vi "show figure (SubVI).vi"(0 "y":bool, 1 "XYGraph引用句柄":refnum<vi>, 2 "文件名长度":i32, 3 "上次的数据列数":i32, 7 "新数据文件":path, 9 "Y输入":refnum<vi>, 12 "X输入":refnum<vi>, 14 "上一次的数据文件":path) -> (4 "figure2datafile输出":path, 6 "数值输出":i32)   [LabVIEW 2019, in "SubVI.lvlib"]
uses:
  SubVI.lvlib
  <vilib>/Utility/miscctls.llb/LVFormatAndPrecisionTypeDef.ctl
  <vilib>/Utility/file.llb/Read Delimited Spreadsheet (DBL).vi
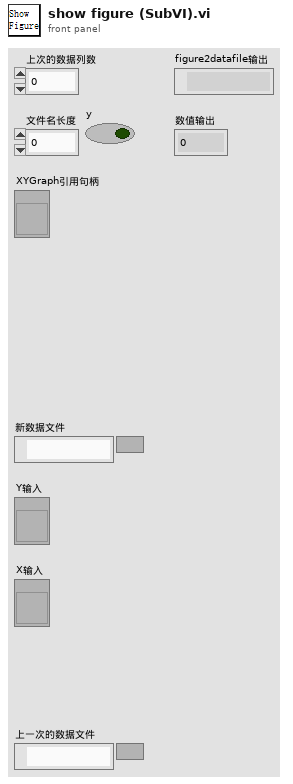
[diagram p1: front panel]
types:
  T1 = typedef "LVFormatAndPrecisionTypeDef.ctl" = cluster{"Format":u8, "Precision":u8}
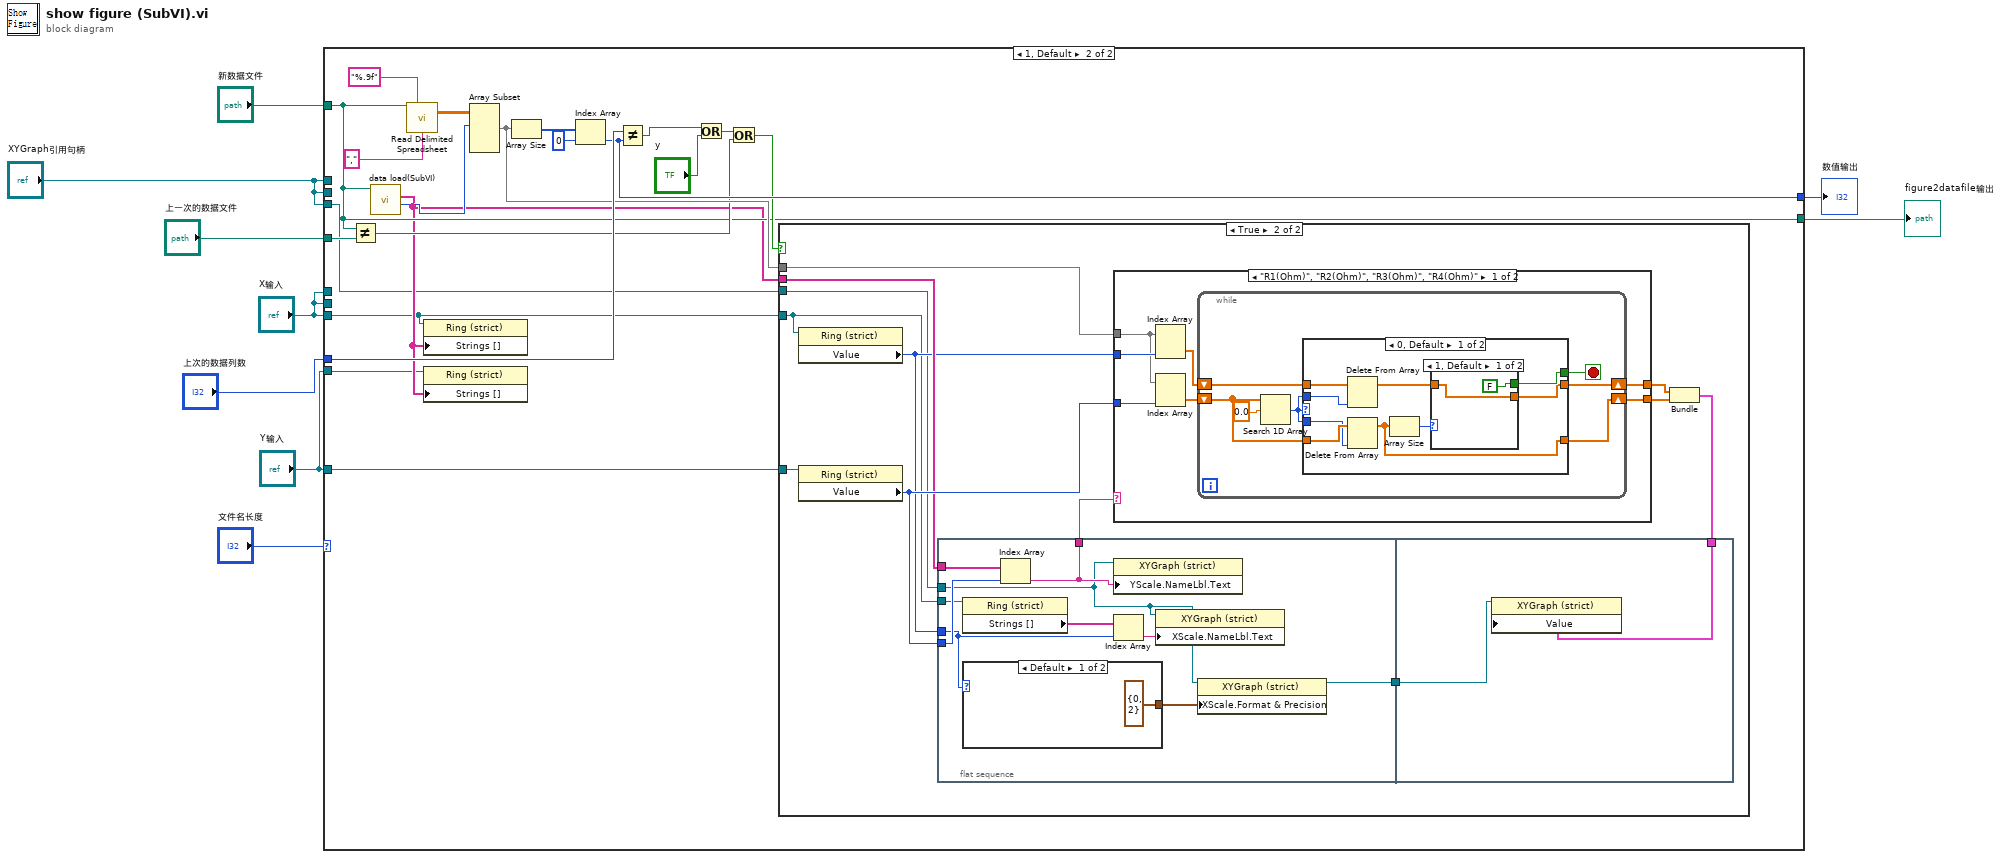
[diagram p0: block diagram]
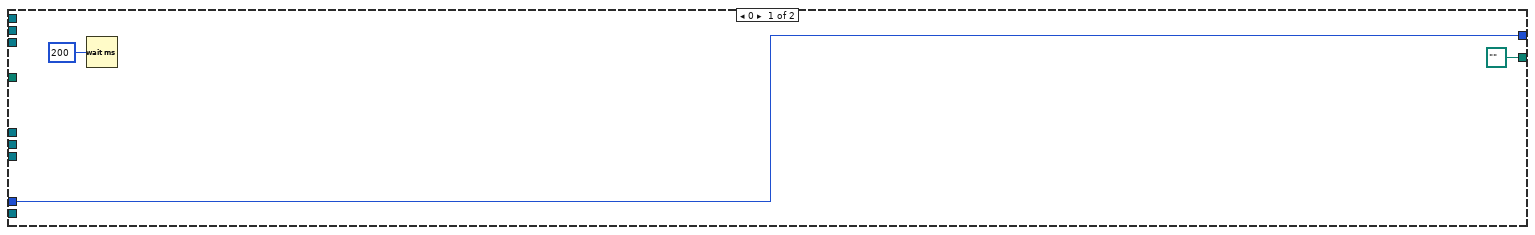
[diagram p2: hidden frame]
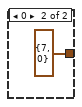
[diagram p4: hidden frame]
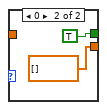
[diagram p5: hidden frame]
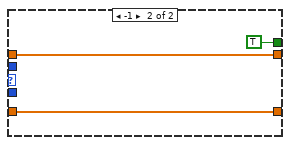
[diagram p6: hidden frame]
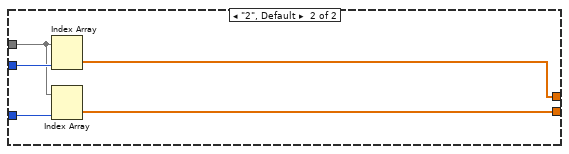
[diagram p7: hidden frame]
diagram:
  n1 = case shown="1, Default" "文件名长度" {
    tunnel: "新数据文件" -> [_ w21]
    tunnel: "上次的数据列数" -> [w12 w28]
    tunnel: [w12 w27] -> w7
    tunnel: "上一次的数据文件" -> [_ w25]
    tunnel: [path "" ("figure2datafile") w21] -> w9
    tunnel: "Y输入" -> [_ w18]
    tunnel: "X输入" -> [_ w14]
    tunnel: "X输入" -> [_ _]
    tunnel: "XYGraph引用句柄" -> [_ _]
    tunnel: "XYGraph引用句柄" -> [_ _]
    tunnel: "XYGraph引用句柄" -> [_ w16]
    tunnel: "X输入" -> [_ _]
    tunnel: "Y输入" -> [_ w15]
    frame 0 {
      n2 = Wait (ms)(milliseconds to wait=u32 200 ("等待时间（毫秒）")) -> ()  [unwired: 1 out]
    }
    frame 1, Default {
      n3 = Not Equal?(x=w21, y=w25) -> (x != y?=w23:bool)
      n4 = call "data load(SubVI).vi"("file path"=w21) -> ("数据起始行"=w20:i32, "项名"=w17:string[])  [unwired: 9 in]
      n5 = call-poly <vilib>:"Read Delimited Spreadsheet.vi"("file path (dialog if empty)"=w21, "format (%.3f)"="%.9f", "delimiter (\\t)"="," ("delimiter (\\t)")) -> ("all rows"=w33:dbl[][])  [unwired: 7 in, 5 out]
      n6 = property on="属性节点" class="Ring (strict)"(reference=w14, "Strings []"=w17) -> ()  [unwired: 1 in, 2 out]
      n7 = property on="属性节点" class="Ring (strict)"(reference=w15, "Strings []"=w17) -> ()  [unwired: 1 in, 2 out]
      n8 = Array Subset(array=w33, index (row)=w20) -> (w26:dbl[][])  [unwired: 3 in]
      n9 = Array Size(array=w26) -> (size(s)=w30:i32[])
      n10 = Index Array(array=w30, index=0 ("索引")) -> (element=w27:i32)
      n11 = Not Equal?(x=w28, y=w27) -> (x != y?=w31:bool)
      n12 = Or(x=w31, y="y") -> (x .or. y?=w24:bool)
      n13 = Or(x=w24, y=w23) -> (x .or. y?=w22:bool)
      n14 = case shown="True" w22 {
        tunnel: w26 -> [_ w42]
        tunnel: w18 -> [_ w40]
        tunnel: w17 -> [_ w38]
        tunnel: w14 -> [_ w35]
        tunnel: w16 -> [_ w36]
        frame False {
        }
        frame True {
          n15 = property class="Ring (strict)"(reference=w35) -> ("Value"=w37:u16)  [unwired: 1 in, 2 out]
          n16 = property class="Ring (strict)"(reference=w40) -> ("Value"=w39:u16)  [unwired: 1 in, 2 out]
          n17 = flat-sequence {
            tunnel: w37 -> [w51]
            tunnel: w39 -> [w52]
            tunnel: [w53] -> w41
            tunnel: w38 -> [w49]
            tunnel: w35 -> [w48]
            tunnel: w36 -> [w47]
            tunnel: [w46] -> w34
            tunnel: w44 -> [w58]
            tunnel: w34 -> [w59]
            frame #0 {
              n18 = property on="属性节点" class="Ring (strict)"(reference=w48) -> ("Strings []"=w55:string[])  [unwired: 1 in, 2 out]
              n19 = case shown="Default" w51 {
                tunnel: [T1 {"Format"=0, "Precision"=2} ("X标尺.显示格式") T1 {"Format"=7, "Precision"=0} ("X标尺.显示格式")] -> w50
                frame Default {
                }
                frame 0 {
                }
              }
              n20 = Index Array(array=w49, index=w52) -> (element=w53:string)
              n21 = property on="属性节点" class="XYGraph (strict)"(reference=w47, "YScale.NameLbl.Text"=w53) -> ()  [unwired: 1 in, 2 out]
              n22 = Index Array(array=w55, index=w51) -> (element=w54:string)
              n23 = property on="属性节点" class="XYGraph (strict)"(reference=w47, "XScale.NameLbl.Text"=w54) -> ()  [unwired: 1 in, 2 out]
              n24 = property on="属性节点" class="XYGraph (strict)"(reference=w47, "XScale.Format & Precision"=w50) -> (reference out=w46:refnum<vi>)  [unwired: 1 in, 1 out]
            }
            frame #1 {
              n25 = property on="属性节点" class="XYGraph (strict)"(reference=w59, "Value"=w58) -> ()  [unwired: 1 in, 2 out]
            }
          }
          n26 = case shown="\"R1(Ohm)\", \"R2(Ohm)\", \"R3(Ohm)\", \"R4(Ohm)\"" w41 {
            tunnel: [w61 w94] -> w45
            tunnel: w39 -> [w66 w93]
            tunnel: w37 -> [w65 w92]
            tunnel: [w60 w91] -> w43
            tunnel: w42 -> [w64 w90]
            frame "R1(Ohm)", "R2(Ohm)", "R3(Ohm)", "R4(Ohm)" {
              n27 = Index Array(array=w64, index (col)=w65) -> (element=w63:dbl[])  [unwired: 1 in]
              n28 = Index Array(array=w64, index (col)=w66) -> (element=w62:dbl[])  [unwired: 1 in]
              n29 = while {
                shift-right: [w70] -> w61
                shift-left: w62 -> [w71]
                shift-right: [w67] -> w60
                shift-left: w63 -> [w69]
                stop <- w72 stop-if-true
                n30 = Search 1D Array(1D array=w71, element=0.0 ("元素")) -> (index of element=w68:i32)  [unwired: 1 in]
                n31 = case shown="0, Default" w68 {
                  tunnel: [w77 TRUE] -> w72
                  tunnel: w71 -> [w82 w87]
                  tunnel: w68 -> [w74 _]
                  tunnel: [w79 w87] -> w70
                  tunnel: w69 -> [w81 w88]
                  tunnel: w68 -> [w80 _]
                  tunnel: [w75 w88] -> w67
                  frame 0, Default {
                    n32 = Delete From Array(array=w81, index=w80) -> (array with subset deleted=w76:dbl[])  [unwired: 1 in, 1 out]
                    n33 = Delete From Array(array=w82, index=w74) -> (array with subset deleted=w79:dbl[])  [unwired: 1 in, 1 out]
                    n34 = Array Size(array=w79) -> (size(s)=w78:i32)
                    n35 = case shown="1, Default" w78 {
                      tunnel: [FALSE TRUE] -> w77
                      tunnel: w76 -> [w83 _]
                      tunnel: [w83 dbl[] []] -> w75
                      frame 1, Default {
                      }
                      frame 0 {
                      }
                    }
                  }
                  frame -1 {
                  }
                }
              }
            }
            frame "2", Default {
              n36 = Index Array(array=w90, index (col)=w92) -> (element=w91:dbl[])  [unwired: 1 in]
              n37 = Index Array(array=w90, index (col)=w93) -> (element=w94:dbl[])  [unwired: 1 in]
            }
          }
          n38 = Bundle(w43, w45) -> (w44:cluster{dbl[], dbl[]})  [unwired: 1 in]
        }
      }
    }
  }
  "figure2datafile输出" <- w9
  "数值输出" <- w7
